vi "Test Controller.vi"(8 "error in":errorcluster) -> ()   [LabVIEW 2025]
doc: "This VI executes continuously carrying out the current operation and responding to updates or new operations. It will often contain the timing or control code that is difficult to place directly in TeleOp. This VI generally opens all sensors and motors and isolates the rest of the robot code from knowing how the operations are carried out."
uses:
  <vilib>/Rock Robotics/WPI/Framework/Completion Status.ctl
  Test Setpoints.ctl
  Test Operations.ctl
  <vilib>/Rock Robotics/WPI/ThirdParty/REV Robotics/REVLib/Typedef/SPARK Feed Forward Gains.ctl
  <vilib>/Rock Robotics/WPI/ThirdParty/REV Robotics/REVLib/Typedef/SPARK PID Gains.ctl
  <vilib>/Rock Robotics/WPI/ThirdParty/REV Robotics/REVLib/Typedef/Spark MAX Control Type.ctl
  <vilib>/Rock Robotics/WPI/ThirdParty/REV Robotics/REVLib/SubVI/Public/SPARK Open Brushless.vi
  <vilib>/Rock Robotics/WPI/ThirdParty/REV Robotics/REVLib/SubVI/Public/SPARK Configure Closed Loop Gains.vi
  <vilib>/Rock Robotics/Network Tables/NT Write Boolean.vi
panel:
  in  "Shooter PID":T1
  in  "Shooter FF":T2={"kV"=0.00185, "kS"=0.0, "kA"=0.0, "kG"=0.0, "kCos"=0.0, "kCosRatio"=0.0}
  in  "Interactive Values":T3
  out "Current\nCmd":string
  in  "Buttons":cluster{"Execute Cmd":bool, "Abort Cmd":bool}
  out "Command Timing":cluster{"Start Time (ms)":u32, "Iterations":i32}
  out "Status":T5
  # "Tip: It may be helpful to observe inputs and sensor values.\nYou may also want to display tuning or debugging controls."
  # "Interactive Command: You may fill in the settings for a command\nand schedule it with the Execute button. You can observe and abort\nany command while fine tuning the code for the controller."
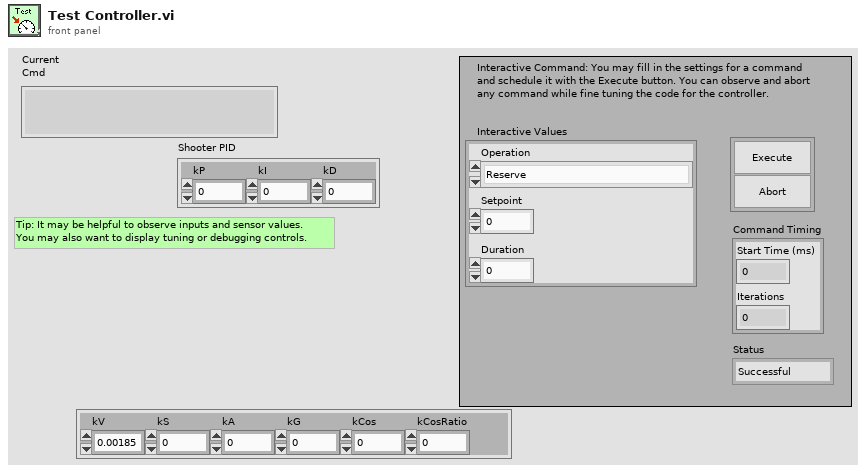
[diagram p1: front panel]
types:
  T1 = typedef "SPARK PID Gains.ctl" = cluster{"kP":dbl, "kI":dbl, "kD":dbl}
  T2 = typedef "SPARK Feed Forward Gains.ctl" = cluster{"kV":dbl, "kS":dbl, "kA":dbl, "kG":dbl, "kCos":dbl, "kCosRatio":dbl}
  T3 = typedef "Test Setpoints.ctl" = cluster{"Operation":T4, "Setpoint":dbl, "Duration":dbl}
  T4 = typedef "Test Operations.ctl" = enum16{"Reserve", "Read Current", "Immediate"}
  T5 = typedef "Completion Status.ctl" = enum16{"Successful", "Aborted", "Incomplete"}
  T6 = typedef "WPI_MotorControlDeviceRef.ctl" = cluster{"DeviceStatus":errorcluster, "Type":T7, "PWM":cluster{"PWM Channel":T8, "DeadBand":T9}, "CAN":cluster{"Device Number":u8, "SetOutput VI Ref":variant, "GetOutput VI Ref":variant, "Enable VI Ref":variant, "Disable VI Ref":variant, "Data":variant}, "Invert":bool, "DIO PWM":cluster{"PWM \"Enable\" Channel":T8, "DIOChannel":T10, "PWM Rate":dbl}}
  T7 = typedef "WPI_MotorControlType.ctl" = enum16{"PWM", "CAN", "DIO PWM"}
  T8 = typedef "FPGA_DIOPWMChannel.ctl" = enum8{"PWM 0", "PWM 1", "PWM 2", "PWM 3", "PWM 4", "PWM 5", "PWM 6", "PWM 7", "PWM 8", "PWM 9", "PWM MXP 0", "PWM MXP 1", "PWM MXP 2", "PWM MXP 3", "PWM MXP 4", "PWM MXP 5", "PWM MXP 6", "PWM MXP 7", "PWM MXP 8", "PWM MXP 9", "Invalid"}
  T9 = typedef "WPI_PWMDeadband.ctl" = cluster{"Name":string, "maxPositivePwm":i32, "minPositivePwm":i32, "centerPwm":i32, "maxNegativePwm":i32, "minNegativePwm":i32, "angularRange":u16}
  T10 = typedef "FPGA_DIOChannel.ctl" = enum8{"DIO 0", "DIO 1", "DIO 2", "DIO 3", "DIO 4", "DIO 5", "DIO 6", "DIO 7", "DIO 8", "DIO 9", "DIO MXP 0", "DIO MXP 1", "DIO MXP 2", "DIO MXP 3", "DIO MXP 4", "DIO MXP 5", "DIO MXP 6", "DIO MXP 7", "DIO MXP 8", "DIO MXP 9", "DIO MXP 10", "DIO MXP 11", "DIO MXP 12", "DIO MXP 13", "DIO MXP 14", "DIO MXP 15", "SPI Port CS1", "SPI Port CS2", "SPI Port CS3", "SPI Port MISO", "SPI Port MOSI", "Invalid"}
  T11 = typedef "Command Status Info.ctl" = cluster{"Name":string, "Status":T5, "notifier out":T12}
  T12 = typedef "Completion Notifier.ctl" = refnum<notifier>
  T13 = cluster{"Current Command":T3, "Command Timing":cluster{"Start Time (ms)":u32, "Iterations":i32}, "Command Arguments":cluster{"Command Info":T11, "Description":string, "Default Command":T3, "queue out":refnum<queue>, "Subsystem Name":string}}
  T14 = typedef "Spark MAX Control Type.ctl" = enum16{"Percent VBus", "Voltage", "Velocity", "Position", "Smart Motion", "Current", "Smart Velocity", "MAXMotion Position", "MAXMotion Velocity"}
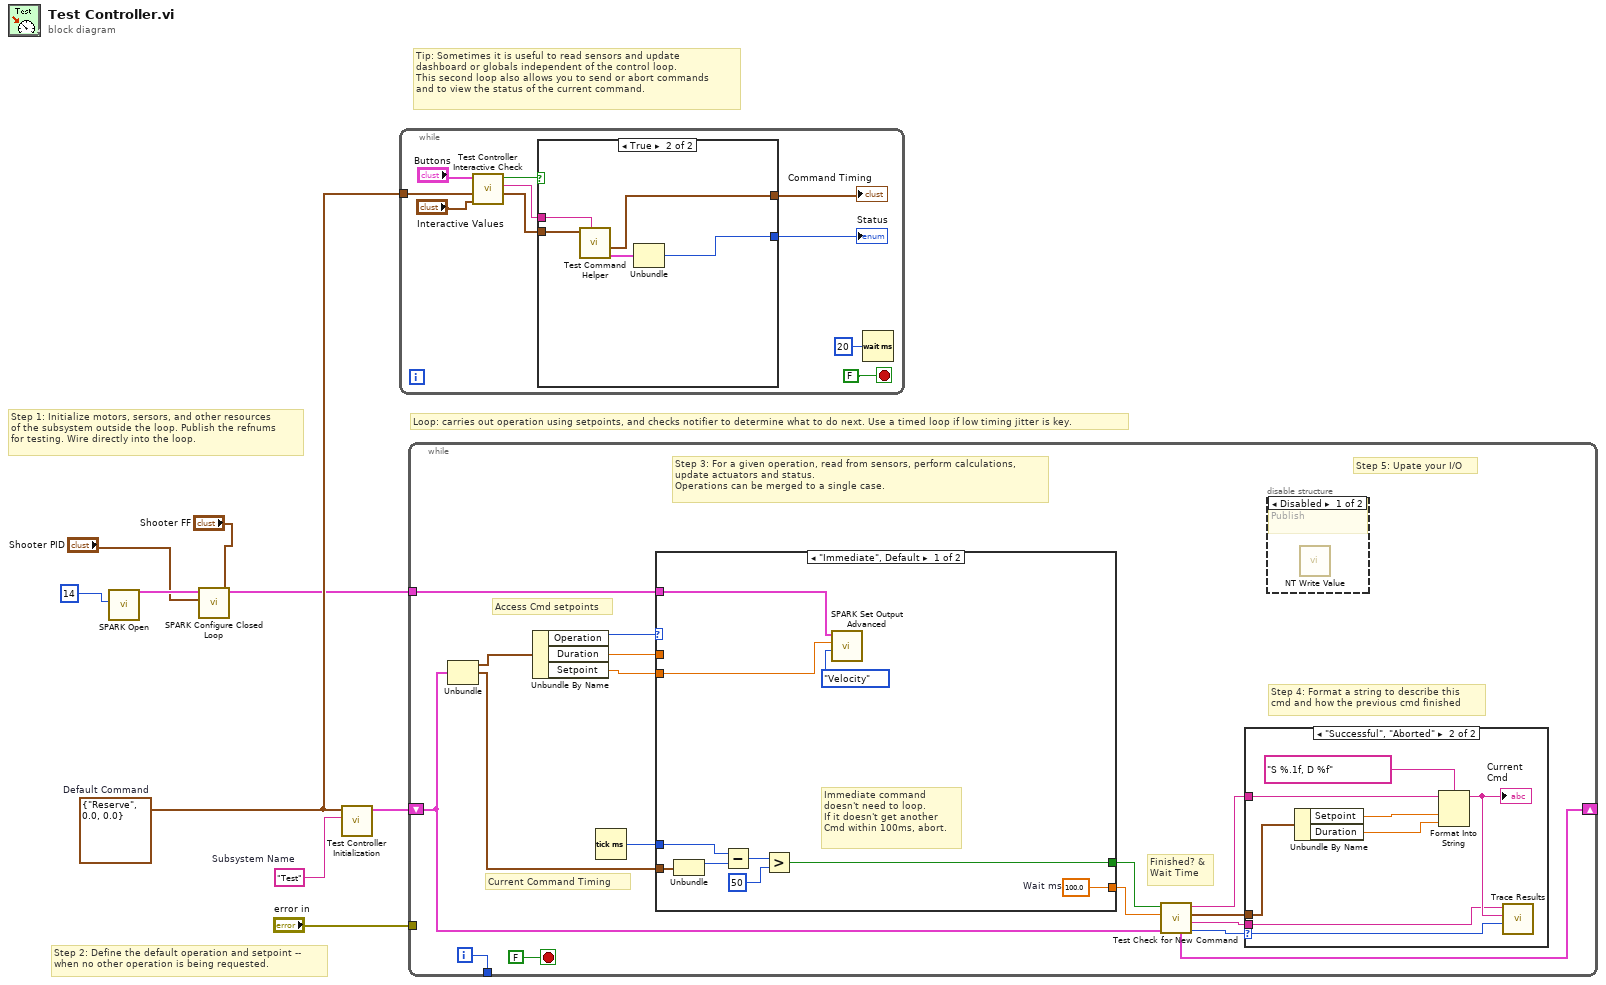
[diagram p0: block diagram]
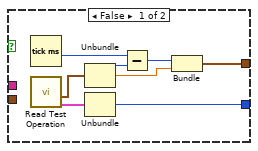
[diagram p2: hidden frame]
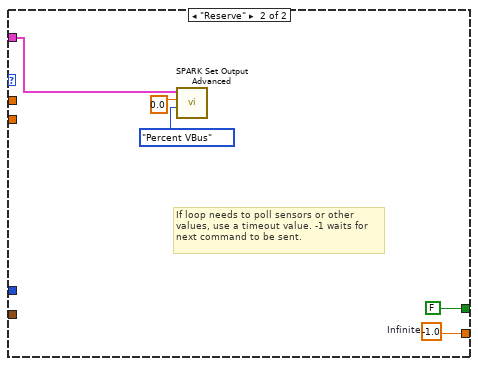
[diagram p5: hidden frame]
diagram:
  w6 = T3 {"Operation"=enum."Reserve", "Setpoint"=0.0, "Duration"=0.0}  # Default Command
  w7 = "Test"  # Subsystem Name
  # "Tip: Sometimes it is useful to read sensors and update\ndashboard or globals independent of the control loop.\nThis second loop also allows you to send or abort commands\nand to view the status of the current command."
  # "Step 2: Define the default operation and setpoint --\nwhen no other operation is being requested."
  # "Step 1: Initialize motors, sersors, and other resources\nof the subsystem outside the loop. Publish the refnums\nfor testing. Wire directly into the loop."
  # "Loop: carries out operation using setpoints, and checks notifier to determine what to do next. Use a timed loop if low timing jitter is key."
  n1 = call-poly <vilib>:"SPARK Open.vi"("Device Number"=u8 14) -> ("MotorControlDeviceRef"=w4:T6)  [unwired: 9 in, 1 out]
  n2 = call-poly <vilib>:"SPARK Configure Closed Loop.vi"("Feed Forward Gains"="Shooter FF", "PID Gains"="Shooter PID", "MotorControlDeviceRef in"=w4) -> ("MotorControlDeviceRef out"=w1:T6)  [unwired: 7 in, 1 out]
  n3 = call "Test Controller Initialization.vi"("Subsystem Name"=w7, "Default Command"=w6) -> ("Current Command"=w8:T13)  [unwired: 9 in]
  n4 = while {
    tunnel: w6 -> [w16]
    stop <- FALSE stop-if-true
    n5 = call "Test Controller Interactive Check.vi"("Interactive Command in"="Interactive Values", "Default Command"=w16, "Buttons"="Buttons") -> ("Interactive Command out"=w13:T3, "Trace String"=w14:string, "Schedule"=w15:bool)  [unwired: 6 in]
    n6 = case shown="True" w15 {
      tunnel: [w27 w32] -> w12
      tunnel: w13 -> [_ w30]
      tunnel: [w23 w28] -> w11
      tunnel: w14 -> [_ w31]
      frame False {
        n7 = Tick Count (ms)() -> (millisecond timer value=w22:u32)
        n8 = call "Read Test Operation.vi"() -> ("Command Info"=w20:T11, "SubSystem Data"=w21:T3)  [unwired: 9 in, 1 out]
        n9 = Unbundle(w21) -> ("Operation"=w26:T4, "Setpoint"=w24:dbl)  [unwired: 1 out]
        n10 = Unbundle(w20) -> ("Status"=w27:T5)  [unwired: 2 out]
        n11 = Subtract(x=w22, y=w26) -> (x-y=w25:u32)
        n12 = Bundle(w25, "Setpoint"=w24) -> (w23:cluster{u32, "Setpoint":dbl})  [unwired: 1 in]
      }
      frame True {
        n13 = call "Test Command Helper.vi"("Description"=w31, "SubSystem Data"=w30) -> ("Command Info Out"=w29:T11, "Command Timing"=w28:cluster{"Start Time (ms)":u32, "Iterations":i32})  [unwired: 7 in, 1 out]
        n14 = Unbundle(w29) -> ("Status"=w32:T5)  [unwired: 2 out]
      }
    }
    "Status" <- w12
    "Command Timing" <- w11
    n15 = Wait (ms)(milliseconds to wait=u32 20) -> ()  [unwired: 1 out]
  }
  n16 = while {
    shift-right: [w41] -> _
    shift-left: w8 -> [w34]
    tunnel: [w48] -> _
    tunnel: "error in" -> [_]
    tunnel: w1 -> [w33]
    i -> [w48]
    stop <- FALSE stop-if-true
    # "Step 5: Upate your I/O"
    # "Step 4: Format a string to describe this\ncmd and how the previous cmd finished"
    # "Current Command Timing"
    # "Access Cmd setpoints"
    # "Finished? &\nWait Time"
    # "Step 3: For a given operation, read from sensors, perform calculations,\nupdate actuators and status.\nOperations can be merged to a single case."
    n17 = Unbundle(w34) -> ("Current Command"=w47:T3, "Command Timing"=w43:cluster{"Start Time (ms)":u32, "Iterations":i32})  [unwired: 1 out]
    n18 = Unbundle By Name(w47) -> ("Operation"=w46:T4, "Duration"=w45:dbl, "Setpoint"=w42:dbl)
    n19 = Tick Count (ms)() -> (millisecond timer value=w44:u32)
    n20 = case shown="\"Immediate\", Default" w46 {
      tunnel: [w67 w72] -> w39
      tunnel: [w61 FALSE ("ignore previous (F)")] -> w40
      tunnel: w43 -> [w63 _]
      tunnel: w45 -> [_ _]
      tunnel: w44 -> [w62 _]
      tunnel: w42 -> [w58 _]
      tunnel: w33 -> [w59 w70]
      frame "Immediate", Default {
        w67 = 100.0  # Wait ms
        # "Immediate command\ndoesn't need to loop.\nIf it doesn't get another\nCmd within 100ms, abort."
        n21 = Unbundle(w63) -> ("Start Time (ms)"=w66:u32)  [unwired: 1 out]
        n22 = Subtract(x=w62, y=w66) -> (x-y=w65:u32)
        n23 = Greater?(x=w65, y=u8 50 ("Left Motor")) -> (0:w61:bool)
        n24 = call <vilib>:"SPARK Set Output Advanced.vi"("Control Mode"=Spark_MAX_Control_Type."Velocity", "Setpoint"=w58, "MotorControlDevRef"=w59) -> ()  [unwired: 7 in, 2 out]
      }
      frame "Reserve" {
        w72 = -1.0  # Infinite
        # "If loop needs to poll sensors or other\nvalues, use a timeout value. -1 waits for\nnext command to be sent."
        n25 = call <vilib>:"SPARK Set Output Advanced.vi"("Control Mode"=Spark_MAX_Control_Type."Percent VBus", "Setpoint"=0.0, "MotorControlDevRef"=w70) -> ()  [unwired: 7 in, 2 out]
      }
    }
    n26 = call "Test Check for New Command.vi"("Current Command"=w34, "Wait time (ms)"=w39, "Finished?"=w40) -> ("Completion"=w35:T5, "Subsystem Name"=w36:string, "Current Command"=w37:T3, "Initial Trace String"=w38:string, "NextCommand"=w41:T13)  [unwired: 4 in]
    n27 = case shown="\"Successful\", \"Aborted\"" w35 {
      selector: w35 -> [_ w57]
      tunnel: w38 -> [_ w53]
      tunnel: w37 -> [_ w54]
      tunnel: w36 -> [_ w50]
      frame "Incomplete", Default {
        # "Continuing current command"
      }
      frame "Successful", "Aborted" {
        # "Report and setup for next command"
        n28 = Unbundle By Name(w54) -> ("Setpoint"=w56:dbl, "Duration"=w51:dbl)
        n29 = Format Into String(format string="S %.1f, D %f", initial string=w53, w56, w51) -> (resulting string=w52:string)  [unwired: 1 in, 1 out]
        "Current\nCmd" <- w52
        n30 = call <vilib>:"Trace Results.vi"("Status of previous command"=w57, "Description"=w52, "Subsystem"=w50) -> ()  [unwired: 9 in]
      }
    }
    n31 = disable-structure shown="Disabled" {
      frame Disabled {
        # "Publish"
        n32 = call-poly <vilib>:"NT Write Value.vi"() -> ()  [unwired: 11 in, 1 out]
      }
      frame Enabled {
      }
    }
  }
